vi "InitialSystem.vi"() -> (0 "error out":errorcluster, 1 "error out 2":errorcluster, 2 "FPGA VI Reference Out":refnum<k20>, 3 "Refnum out":refnum<k21>)   [LabVIEW 2017]
uses:
  <vilib>/rvi/interface/nirviOpenFPGA/nirviOpenFPGA.xnode
  FPGA Bitfiles/TrustFFPert_FPGATarget_FPGAMotorControl_c8r18+Kz+j0.lvbitx
  <vilib>/FPGAPlugInAG/PXI-7842R/niLvFpga_Open_PXI-7842R.vi
  FPGA/FPGA_MotorControl.vi
  <vilib>/rvi/interface/common/dynamic/niFpgaDynamicAddResources.vi
  <vilib>/rvi/interface/nirviMethod/nirviMethod.xnode
  <vilib>/FPGAPlugInAG/Dynamic/niLvFpga_Run_Dynamic.vi
  <vilib>/FPGAPlugInAG/Dynamic/niLvFpga_Reset_Dynamic.vi
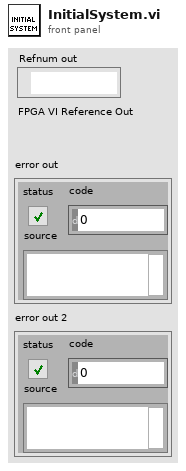
[diagram p1: front panel]
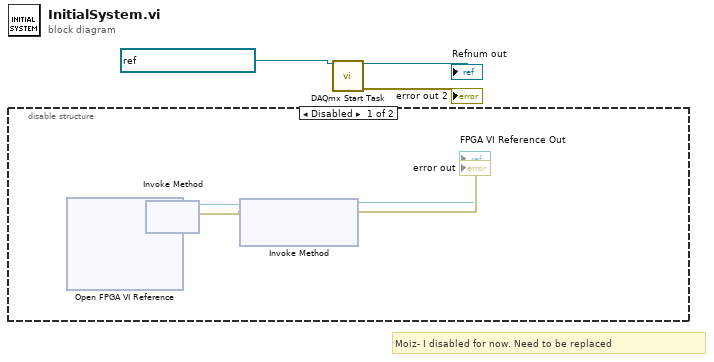
[diagram p0: block diagram]
diagram:
  # "Moiz- I disabled for now. Need to be replaced"
  n1 = disable-structure shown="Disabled" {
    frame Disabled {
      n2 = xnode "Open FPGA VI Reference"() -> ("FPGA VI Reference Out"=w4:refnum<k20>, "error out"=w5:errorcluster)  [unwired: 2 in]
      n3 = xnode "Invoke Method"("FPGA VI Reference In"=w4, "error in"=w5) -> ("FPGA VI Reference Out"=w6:refnum<k20>, "error out"=w7:errorcluster)
      n4 = xnode "Invoke Method"("FPGA VI Reference In"=w6, "error in"=w7) -> ("FPGA VI Reference Out"=→"FPGA VI Reference Out":refnum<k20>, "error out"=→"error out":errorcluster)  [unwired: 1 in]
    }
    frame Enabled {
    }
  }
  n5 = call <vilib>:"DAQmx Start Task.vi"("task/channels in"=refnum<k21> "TensionSens239" ("DAQmx Task Name")) -> ("task out"=→"Refnum out":refnum<k21>, "error out"=→"error out 2":errorcluster)  [unwired: 13 in]
